vi "Main.vi"() -> ()   [LabVIEW 2019]
uses:
  Status.ctl
  Command.ctl
  <extravilib>/ChannelInstances/MessengerM-t'Command.ctl'/Write With Abort.vi
  <extravilib>/ChannelInstances/Messenger-c(i32,t'Status.ctl')/Read With Abort.vi
  <resource>/Channels/Messenger/Read With Abort.vi
  <vilib>/ChannelSupport/Channel Message/Read ID.vi
  <extravilib>/ChannelInstances/Messenger-c(i32,t'Status.ctl')/Instantiate.vi
  <resource>/Channels/Messenger/Endpoint.vi
  <extravilib>/ChannelInstances/Messenger-c(i32,t'Status.ctl')/Unwrap.vi
  <extravilib>/ChannelInstances/MessengerM-t'Command.ctl'/Instantiate.vi
  <extravilib>/ChannelInstances/MessengerM-t'Command.ctl'/Endpoint.vi
  <extravilib>/ChannelInstances/MessengerM-t'Command.ctl'.lvlib
  <extravilib>/ChannelInstances/Messenger-c(i32,t'Status.ctl').lvlib
panel:
  in  "exit":bool
  in  "command":T1
  out "status":T2[](array[typedef]) items=["exited", "off", "active", "standby", "error"]
  in  "active station":enum32{"0", "1", "2", "3", "4", "5", "6", "7"}(radio)
  in  "send":bool
  # "select station, select command, send"
  # "station"
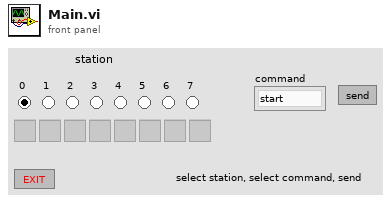
[diagram p1: front panel]
types:
  T1 = typedef "Command.ctl" = enum16{"start", "stop", "pause", "resume", "reset", "exit"}
  T2 = typedef "Status.ctl" = u16
  T3 = typedef "MessengerM-t'Command.ctl'.lvlib/))Channel.ctl" = refnum<queue>
  T4 = typedef "Messenger-c(i32,t'Status.ctl').lvlib/))Channel.ctl" = refnum<queue>
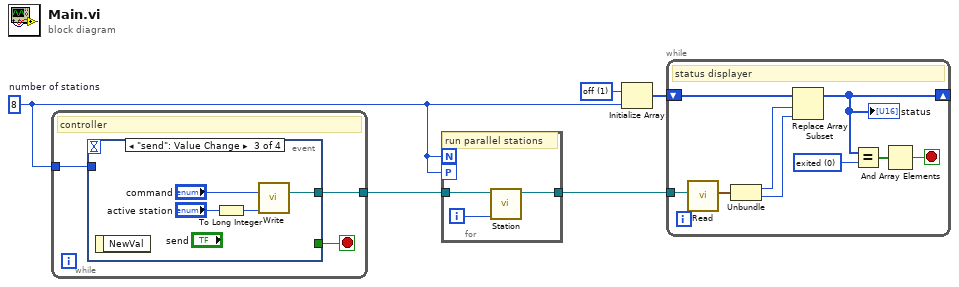
[diagram p0: block diagram]
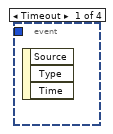
[diagram p2: hidden frame]
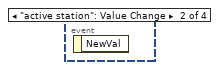
[diagram p3: hidden frame]
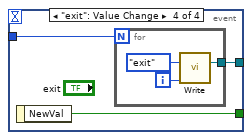
[diagram p4: hidden frame]
diagram:
  w3 = T2 1 items=["exited", "off", "active", "standby", "error"] ("status")
  w1 = 8  # number of stations
  n1 = while {
    tunnel: [w8] -> w5
    tunnel: w1 -> [w6]
    stop <- w7 stop-if-true
    # "controller"
    n2 = event shown="[2] \"send\": Value Change" {
      selector: _ -> [_ _ _ _]
      dyn-events: _ -> [_ _ _ _]
      timeout: _ -> [_ _ _ _]
      tunnel: [_ _ w10 w14] -> w8
      tunnel: [_ _ _ w15] -> w7
      tunnel: w6 -> [_ _ _ w13]
      event Timeout {
        n3 = event-data() -> ()  [unwired: 1 in, 3 out]
      }
      event "active station": Value Change {
        n4 = event-data() -> ()  [unwired: 1 in, 1 out]
      }
      event "send": Value Change {
        n5 = event-data() -> ()  [unwired: 1 in, 1 out]
        n6 = To Long Integer(number="active station") -> (32bit integer=w11:i32)
        n7 = call <extravilib>:"Write.vi"("element"="command", "subchannel (0)"=w11) -> ("channel"=w10:T3)  [unwired: 10 in, 3 out]
      }
      event "exit": Value Change {
        n8 = event-data() -> ("NewVal"=w15:bool)  [unwired: 1 in]
        n9 = for {
          N: w13 -> [_]
          tunnel: [w18] -> w14
          i -> [w17]
          n10 = call <extravilib>:"Write.vi"("element"=Command."exit", "subchannel (0)"=w17) -> ("channel"=w18:T3)  [unwired: 10 in, 3 out]
        }
      }
    }
  }
  n11 = for {
    N: w1 -> [_]
    tunnel: w5 -> [w21]
    workers-P: w1 -> [_]
    tunnel: [w20] -> w4
    i -> [w19]
    # "run parallel stations"
    n12 = call "Station.vi"("station #"=w19, "command"=w21) -> ("status"=w20:T4)  [unwired: 9 in]
  }
  n13 = Initialize Array(w3, w1) -> (w2:T2[])
  n14 = while {
    tunnel: w4 -> [w30]
    shift-right: [w25] -> _
    shift-left: w2 -> [w28]
    stop <- w23 stop-if-true
    w22 = T2 0 items=["exited", "off", "active", "standby", "error"] ("status")
    # "status displayer"
    n15 = call <extravilib>:"Read.vi"("channel"=w30) -> ("element"=w29:cluster{"station #":i32, "status":T2})  [unwired: 7 in, 3 out]
    n16 = Unbundle(w29) -> ("station #"=w27:i32, "status"=w26:T2)
    n17 = Replace Array Subset(array=w28, new element=w26, index=w27) -> (w25:T2[])
    "status" <- w25
    n18 = Equal?(x=w25, y=w22) -> (x = y?=w24:bool[])
    n19 = And Array Elements(Boolean array=w24) -> (logical AND=w23:bool)
  }
